vi "Main_System.vi"(7 "LabVIEW Web Service Request":refnum<class "Web Request.lvclass">) -> ()   [LabVIEW 2017]
uses:
  <vilib>/wsapi/Web Request.lvclass
  SubVIs/System_States.ctl
panel:
  in  "Tab Control":enum32{"Page 1", "Page 2"}(tab)
  out "error IO":errorcluster
  out "JSON string":string
  out "Next State":T1
  out "Output/Debug":T2={"Test_File"="", "Status"="OK", "RF_Center_Freq"="0", "RF_Gain"="0", "BB_Gain"="0", "Error"=""}
  out "This State":T1
  in  "View TDMS Header information":bool
  in  "Enable scaling":bool=TRUE
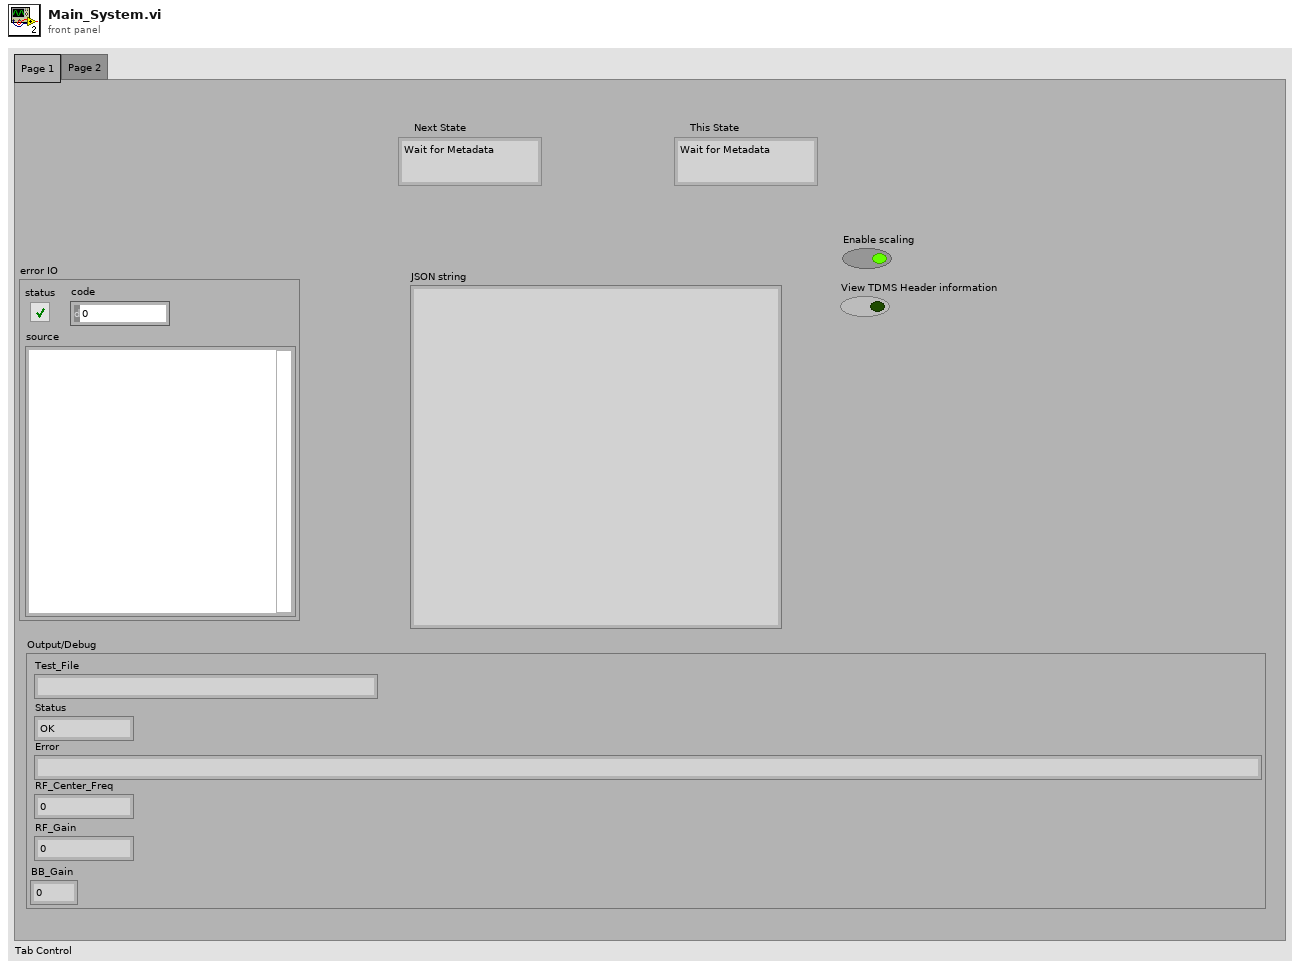
[diagram p1: front panel]
types:
  T1 = typedef "System_States.ctl" = enum16{"Wait for Metadata", "Parse Metadata", "Play File", "Finished Playing", "Send Message", "Report Error", "Exit"}
  T2 = cluster{"Test_File":string, "Status":string, "RF_Center_Freq":string, "RF_Gain":string, "BB_Gain":string, "Error":string}
  T3 = cluster{"Test_File":string, "Status":string, "RF_Center_Freq":string, "RF_Gain":string, "BB_Gain":string, "Error 2":string}
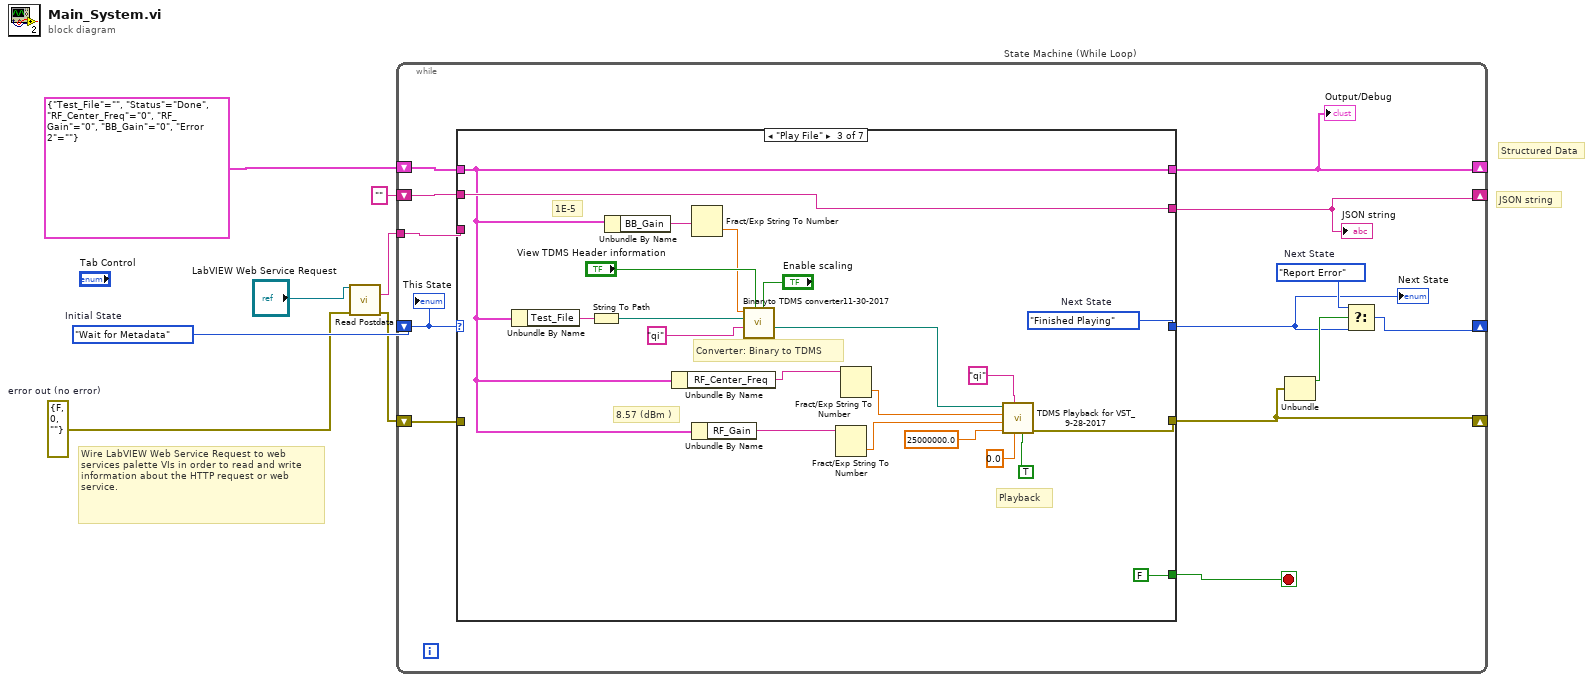
[diagram p0: block diagram]
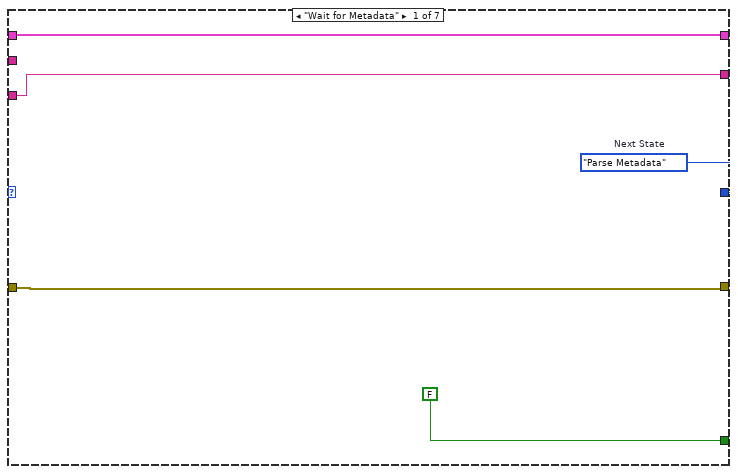
[diagram p2: hidden frame]
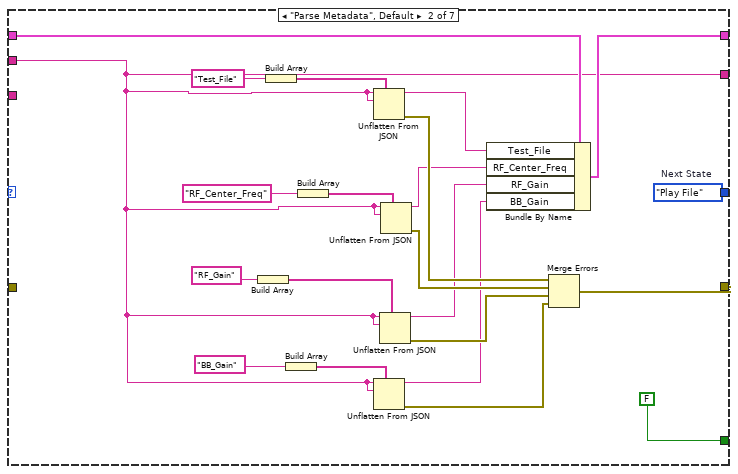
[diagram p3: hidden frame]
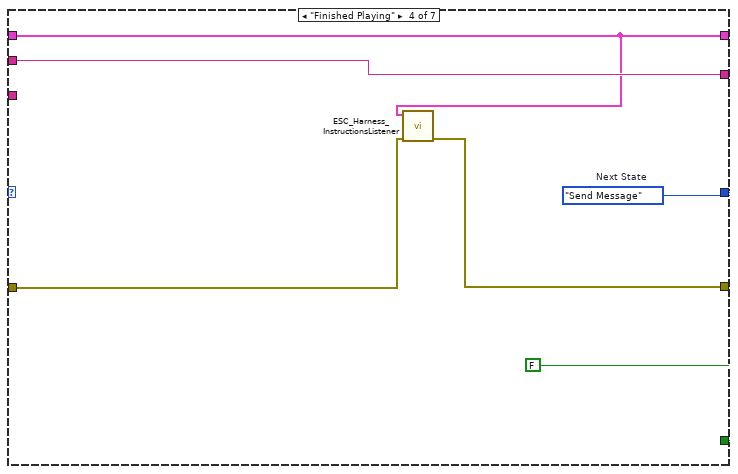
[diagram p4: hidden frame]
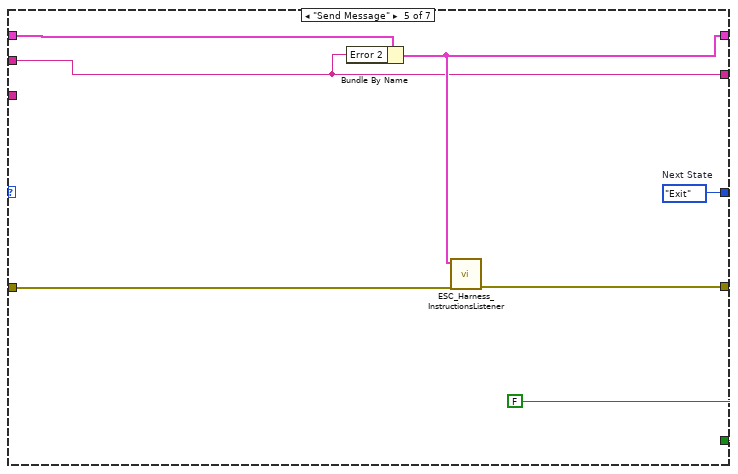
[diagram p5: hidden frame]
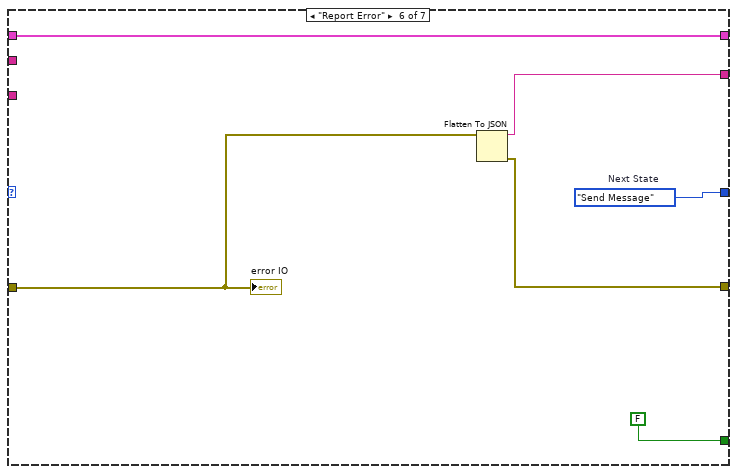
[diagram p6: hidden frame]
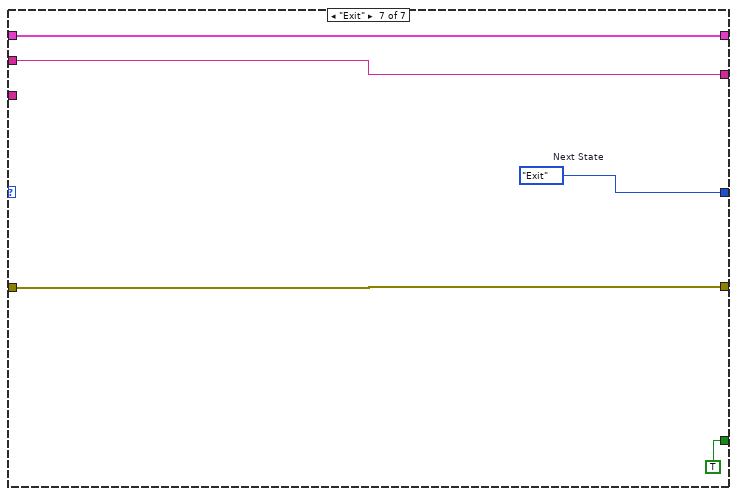
[diagram p7: hidden frame]
diagram:
  w5 = errorcluster {"status"=FALSE, "code"=0, "source"=""}  # error out (no error)
  w7 = System_States."Wait for Metadata"  # Initial State
  # "Wire LabVIEW Web Service Request to web services palette VIs in order to read and write information about the HTTP request or web service."
  # "JSON string"
  # "Structured Data"
  n1 = call <vilib>:"Read Postdata.vi"("LabVIEW Web Service Request"="LabVIEW Web Service Request", "error in (no error)"=w5) -> ("postdata"=w2:string, "error out"=w4:errorcluster)  [unwired: 11 in, 1 out]
  n2 = while "State Machine (While Loop)" {
    shift-right: [w17] -> _
    shift-left: w7 -> [w8]
    shift-right: [w13] -> _
    shift-left: "" ("JSON string") -> [w19]
    shift-right: [w9] -> _
    shift-left: T3 {"Test_File"="", "Status"="Done", "RF_Center_Freq"="0", "RF_Gain"="0", "BB_Gain"="0", "Error 2"=""} -> [w18]
    shift-right: [w16] -> _
    shift-left: w4 -> [w14]
    tunnel: w2 -> [w10]
    stop <- w20 stop-if-true
    w12 = System_States."Report Error"  # Next State
    n3 = case shown="\"Play File\"" w8 {
      tunnel: [FALSE FALSE FALSE FALSE FALSE FALSE TRUE] -> w20
      tunnel: [w24 w37 w68 w73 w80 w86 w91] -> w11
      tunnel: w19 -> [_ w28 w67 w72 w76 _ w90]
      tunnel: w18 -> [w23 w40 w59 w69 w78 w82 w89]
      tunnel: [w23 w38 w59 w69 w77 w82 w89] -> w9
      tunnel: [w21 w28 w67 w72 w76 w83 w90] -> w13
      tunnel: [w22 w33 w63 w70 w75 w85 w88] -> w16
      tunnel: w14 -> [w22 _ _ w71 w81 w84 w88]
      tunnel: w10 -> [w21 _ _ _ _ _ _]
      frame "Wait for Metadata" {
        w24 = System_States."Parse Metadata"  # Next State
      }
      frame "Parse Metadata", Default {
        w37 = System_States."Play File"  # Next State
        n4 = Build Array("RF_Gain") -> (w43:string[])
        n5 = Build Array("Test_File") -> (w41:string[])
        n6 = Build Array("BB_Gain") -> (w29:string[])
        n7 = Build Array("RF_Center_Freq") -> (w42:string[])
        n8 = Unflatten From JSON(path=w41, JSON string=w28, type and defaults=w28) -> (value=w39:string, error out=w36:errorcluster)  [unwired: 4 in]
        n9 = Unflatten From JSON(path=w29, JSON string=w28, type and defaults=w28) -> (value=w26:string, error out=w27:errorcluster)  [unwired: 4 in]
        n10 = Unflatten From JSON(path=w43, JSON string=w28, type and defaults=w28) -> (value=w31:string, error out=w34:errorcluster)  [unwired: 4 in]
        n11 = Unflatten From JSON(path=w42, JSON string=w28, type and defaults=w28) -> (value=w32:string, error out=w35:errorcluster)  [unwired: 4 in]
        n12 = Bundle By Name(cluster=w40, "Test_File"=w39, "RF_Center_Freq"=w32, "RF_Gain"=w31, "BB_Gain"=w26) -> (w38:T3)
        n13 = Merge Errors(w36, w35, w34, w27) -> (w33:errorcluster)
      }
      frame "Play File" {
        w68 = System_States."Finished Playing"  # Next State
        # "Playback"
        # "Converter: Binary to TDMS"
        # "8.57 (dBm )"
        # "1E-5"
        n14 = Unbundle By Name(w59) -> ("Test_File"=w64:string)
        n15 = String To Path(string=w64) -> (path=w58:path)
        n16 = Unbundle By Name(w59) -> ("BB_Gain"=w53:string)
        n17 = Unbundle By Name(w59) -> ("RF_Center_Freq"=w52:string)
        n18 = Fract/Exp String To Number(string=w53) -> (number=w49:dbl)  [unwired: 3 in, 1 out]
        n19 = Unbundle By Name(w59) -> ("RF_Gain"=w65:string)
        n20 = call "Binaryto TDMS converter11-30-2017.vi"("Label header with scale information (on/ OFF)"="Enable scaling", "View TDMS Header information (on/ off)"="View TDMS Header information", "channel name"="qi", "original binary file Location"=w58, "Scale Data"=w49) -> ("Converted Binary to TDMS location"=w54:path)  [unwired: 6 in]
        n21 = Fract/Exp String To Number(string=w65) -> (number=w57:dbl)  [unwired: 3 in, 1 out]
        n22 = Fract/Exp String To Number(string=w52) -> (number=w51:dbl)  [unwired: 3 in, 1 out]
        n23 = call "TDMS Playback for VST_9-28-2017.vi"("IQ Swap Enabled"=TRUE, "pre filter gain"=0.0, "channel name (iq/qi)"="qi", "IQ Rate (S/s)"=25000000.0, "Output Power (dBm)"=w57, "Carrier (Hz)"=w51, "Path"=w54) -> ("error out"=w63:errorcluster)  [unwired: 4 in]
      }
      frame "Finished Playing" {
        w73 = System_States."Send Message"  # Next State
        n24 = call "ESC_Harness_InstructionsListener.vi"("error in (no error)"=w71, "Input"=w69) -> ("error out"=w70:errorcluster)  [unwired: 8 in]
      }
      frame "Send Message" {
        w80 = System_States."Exit"  # Next State
        n25 = Bundle By Name(cluster=w78, "Error 2"=w76) -> (w77:T3)
        n26 = call "ESC_Harness_InstructionsListener.vi"("error in (no error)"=w81, "Input"=w77) -> ("error out"=w75:errorcluster)  [unwired: 8 in]
      }
      frame "Report Error" {
        w86 = System_States."Send Message"  # Next State
        n27 = Flatten To JSON(anything=w84) -> (JSON string=w83:string, 11:w85:errorcluster)  [unwired: 2 in]
        "error IO" <- w84
      }
      frame "Exit" {
        w91 = System_States."Exit"  # Next State
      }
    }
    "JSON string" <- w13
    "Next State" <- w11
    "Output/Debug" <- w9
    n28 = Unbundle(w16) -> ("status"=w15:bool)  [unwired: 2 out]
    n29 = Select(t=w12, s=w15, f=w11) -> (s? t:f=w17:T1)
    "This State" <- w8
  }
